vi "Angle-Agle synergy.vi"(11 "Angle for Synergy analysis":dbl[][](array[numeric])) -> (2 "Angle-angle synergygrap":i32[][](array[numeric]), 3 "Angle-angle synergy":dbl[][](array[numeric]))   [LabVIEW 2020]
uses:
  <vilib>/Analysis/NI_AALPro.lvlib
  <vilib>/gmath/NI_Gmath.lvlib
panel:
  out "Angle-angle synergy graph":i32[][](array[numeric])
  out "Angle-angle synergy":dbl[](array[numeric])
  out "r^2":dbl format="%.7g"
  out "correlation coefficient r":dbl format="%.7g"
  out "Elbow flexion - Shoulder graph":i32[](graph)
  out "Elbow flexion - Shoulder extension %":i32
  out "Elbow flexion - Shoulder flexion %":i32
  out "Shoulder flexion - Elbow graph":i32[](graph)
  out "Shoulder flexion - Elbow extension %":i32
  out "Shoulder flexion - Elbow flexion %":i32
  out "Elbow flexion tags":i32[](array[numeric])
  out "Shoulder flexion tags":i32[](array[numeric])
  out "Elbow extension - Shoulder graph":i32[](graph)
  out "Elbow extension - Shoulder flexion %":i32
  out "Elbow extension- Shoulder extension %":i32
  out "Shoulder extension - Elbow graph":i32[](graph)
  out "Shoulder extension - Elbow flexion %":i32
  out "Shoulder extension- Elbow extension %":i32
  out "Shoulder derivative":dbl[](graph)
  out "Shoulder":dbl[](graph)
  out "Shoulder to derivate":dbl[](array[numeric])
  out "Wrist X to graph":dbl[](array[numeric])
  out "Elbow extension tags":i32[](array[numeric])
  out "Shoulder extension tags":i32[](array[numeric])
  out "?":dbl[](graph)
  out "?":dbl[](graph)
  # "Elbow"
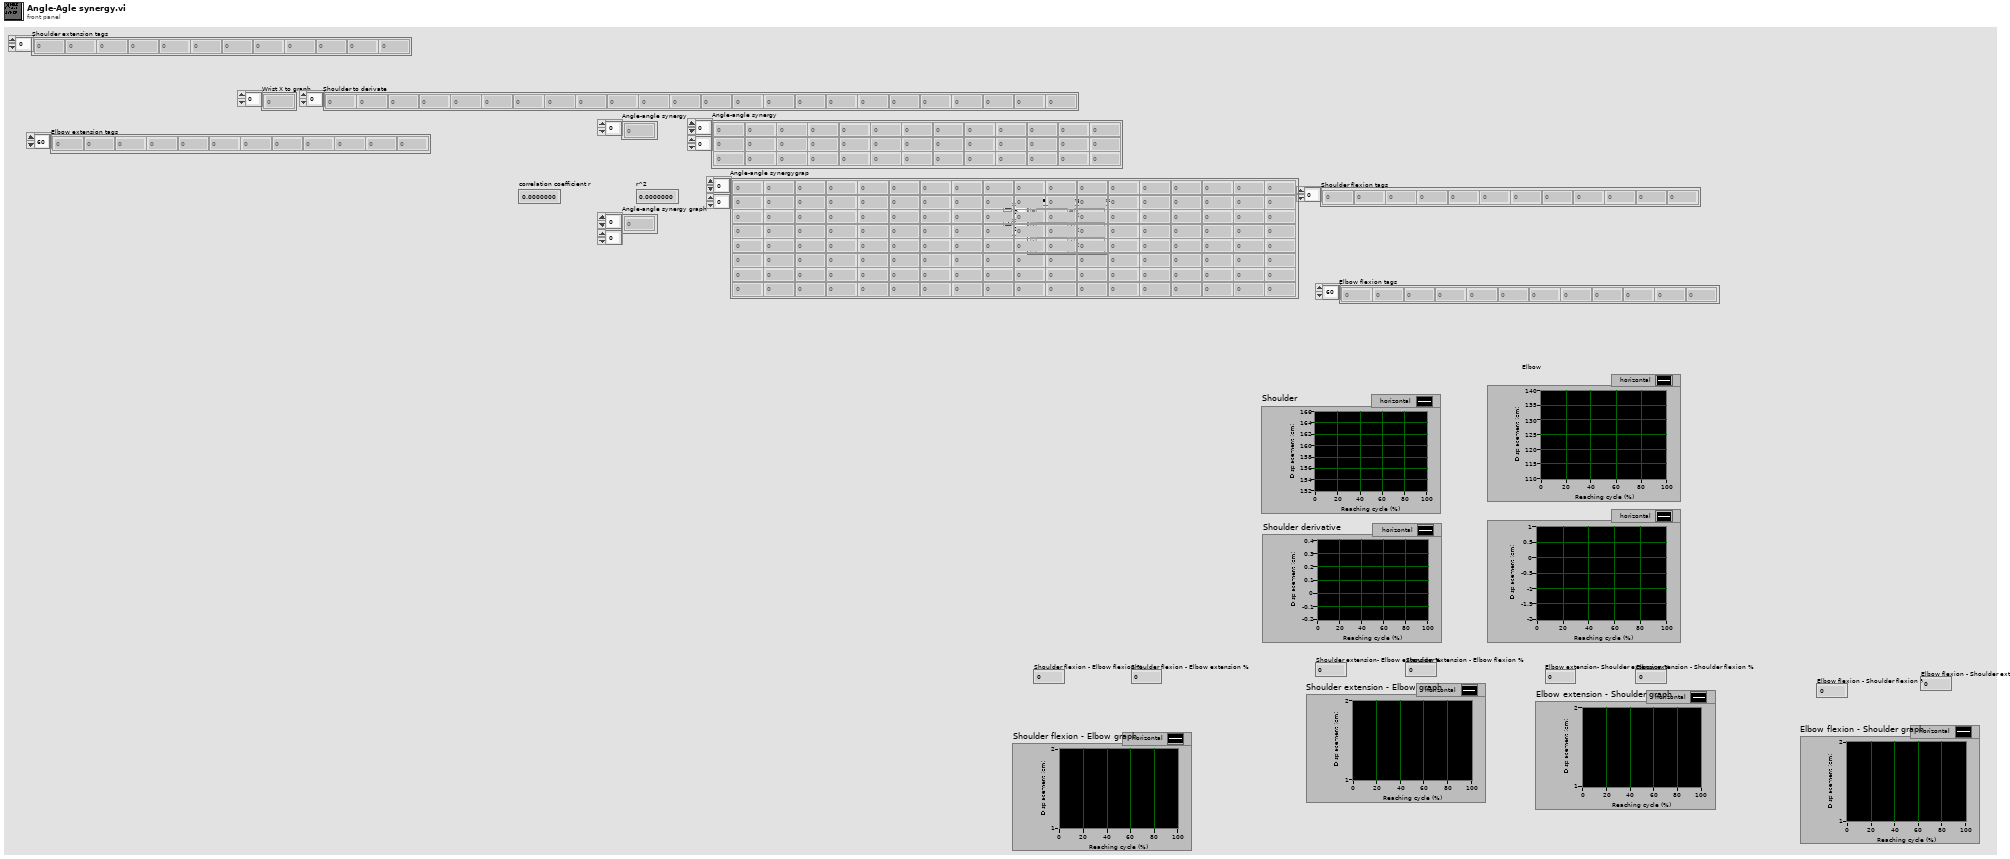
[diagram p1: front panel]
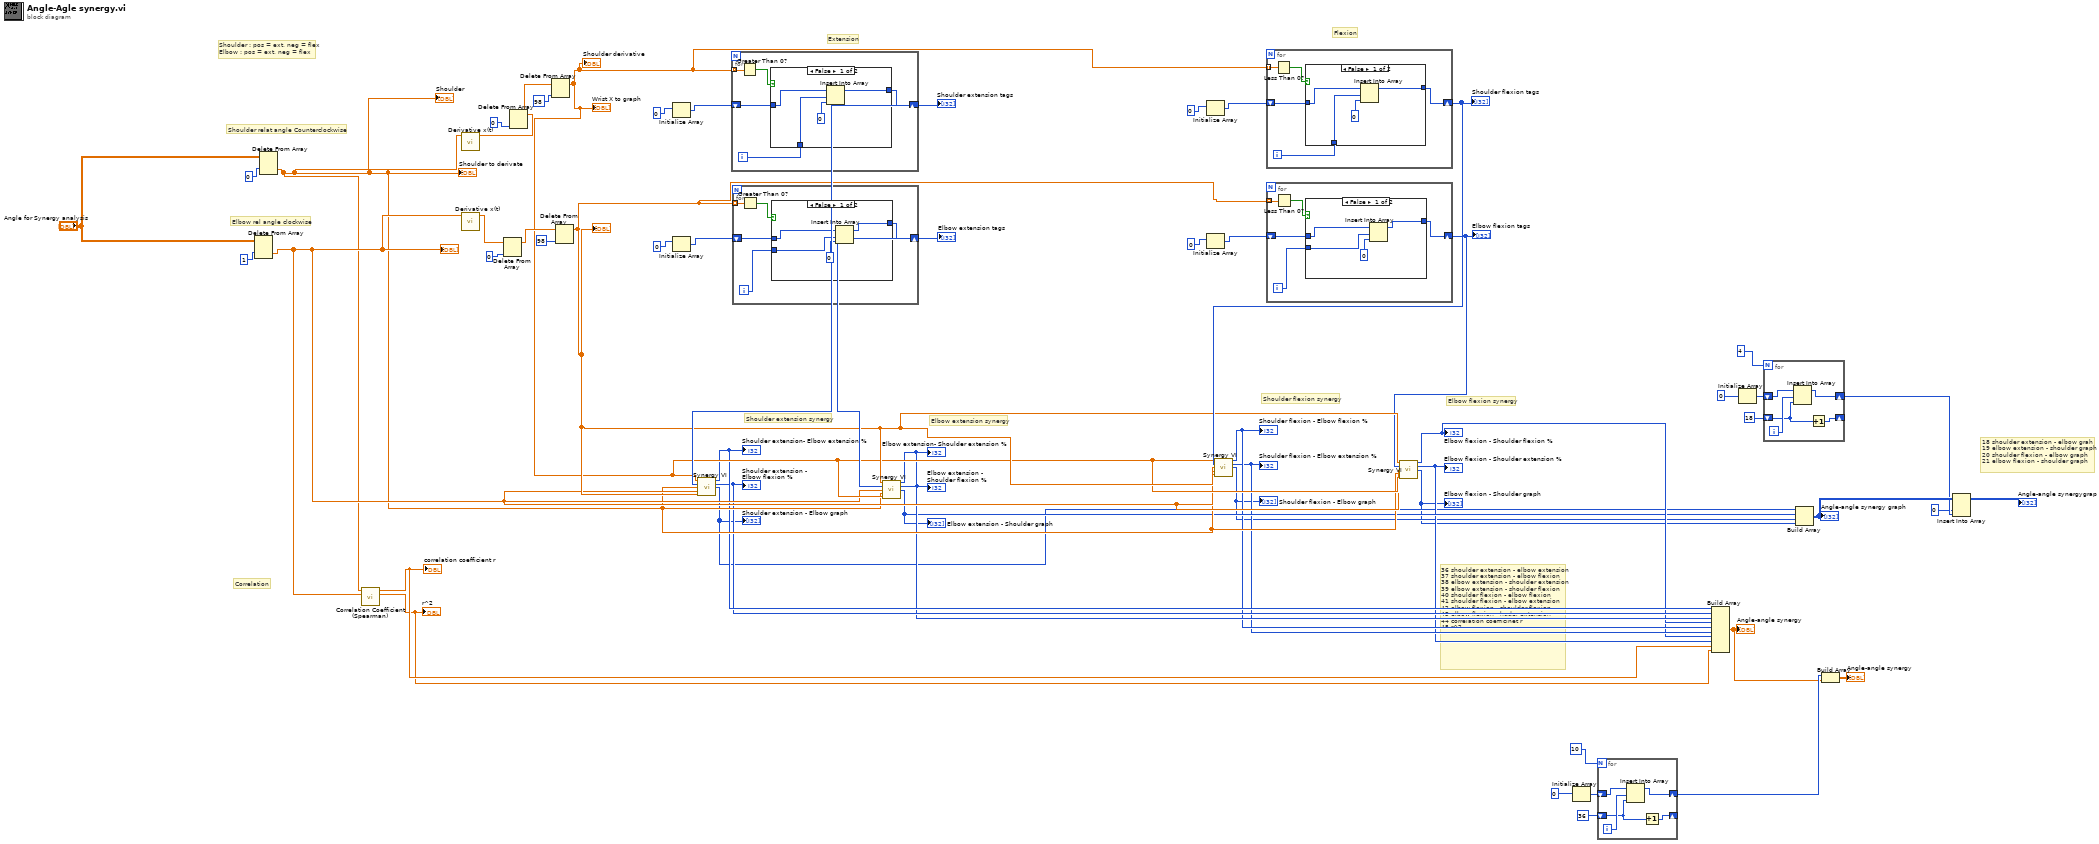
[diagram p0: block diagram]
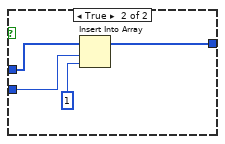
[diagram p2: hidden frame]
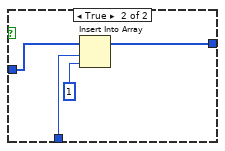
[diagram p3: hidden frame]
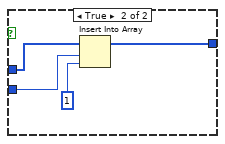
[diagram p4: hidden frame]
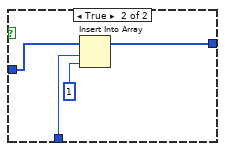
[diagram p5: hidden frame]
diagram:
  # "18 shoulder extension - elbow grah\n19 elbow extension - shoulder graph\n20 shoulder flexion - elbow graph\n21 elbow flexion - shoulder graph"
  # "36 shoulder extension - elbow extension\n37 shoulder extension - elbow flexion\n38 elbow extension - shoulder extension\n39 elbow extension - shoulder flexion\n40 shoulder flexion - elbow flexion\n41 shoulder flexion - elbow extension\n42 elbow flexion - shoulder flexion\n43 elbow flexion - huder extension\n44 correlation coefficinet r\n45 r^2"
  # "Correlation"
  # "Elbow flexion synergy"
  # "Shoulder flexion synergy"
  # "Flexion"
  # "Extension"
  # "Elbow extension synergy"
  # "Shoulder extension synergy"
  # "Shoulder : pos = ext, neg = flex\nElbow : pos = ext, neg = flex"
  # "Elbow rel angle clockwise"
  # "Shoulder relat angle Counterclockwise"
  n1 = Delete From Array(array="Angle for Synergy analysis", index (row)=1) -> (deleted portion=w31:dbl[])  [unwired: 2 in, 1 out]
  "?" <- w31
  n2 = Delete From Array(array="Angle for Synergy analysis", index (row)=0) -> (deleted portion=w30:dbl[])  [unwired: 2 in, 1 out]
  "Shoulder to derivate" <- w30
  "Shoulder" <- w30
  n3 = call <vilib>:"Correlation Coefficient (Spearman).vi"("Y"=w31, "X"=w30) -> ("r^2"=w20:dbl, "correlation coefficient r"=w21:dbl)  [unwired: 8 in]
  "correlation coefficient r" <- w21
  "r^2" <- w20
  n4 = call <vilib>:"Derivative x(t).vi"("X"=w30) -> ("dX/dt"=w56:dbl[])  [unwired: 9 in, 1 out]
  n5 = call <vilib>:"Derivative x(t).vi"("X"=w31) -> ("dX/dt"=w49:dbl[])  [unwired: 9 in, 1 out]
  n6 = Delete From Array(array=w49, index=0) -> (array with subset deleted=w50:dbl[])  [unwired: 1 in, 1 out]
  n7 = Delete From Array(array=w56, index=0) -> (array with subset deleted=w53:dbl[])  [unwired: 1 in, 1 out]
  n8 = Delete From Array(array=w53, index=98) -> (array with subset deleted=w32:dbl[])  [unwired: 1 in, 1 out]
  "Wrist X to graph" <- w32
  "Shoulder derivative" <- w32
  n9 = Delete From Array(array=w50, index=98) -> (array with subset deleted=w34:dbl[])  [unwired: 1 in, 1 out]
  "?" <- w34
  n10 = Initialize Array(0) -> (w47:i32[])  [unwired: 1 in]
  n11 = Initialize Array(0) -> (w45:i32[])  [unwired: 1 in]
  n12 = for {
    tunnel: w32 -> [w61] mode=indexing
    shift-right: [w58] -> w41
    shift-left: w47 -> [w59]
    i -> [w57]
    n13 = Greater Than 0?(x=w61) -> (x > 0?=w60:bool)
    n14 = case shown="False" w60 {
      tunnel: w59 -> [w64 w69]
      tunnel: [w63 w68] -> w58
      tunnel: w57 -> [w62 w66]
      frame False {
        n15 = Insert Into Array(array=w64, index=w62, new element=0) -> (w63:i32[])
      }
      frame True {
        n16 = Insert Into Array(array=w69, index=w66, new element=1) -> (w68:i32[])
      }
    }
  }
  "Shoulder extension tags" <- w41
  n17 = call "Synergy VI.vi"("Wrist X to graph"=w32, "Wrist X Tags"=w41, "Wrist X to derivate"=w30, "Shoulder X to derivate"=w31, "Shoulder X"=w34) -> ("same direction %"=w29:i32, "opposite direction %"=w28:i32, "WristX-ShouldeX graph"=w12:i32[])  [unwired: 8 in]
  "Shoulder extension- Elbow extension %" <- w29
  "Shoulder extension - Elbow flexion %" <- w28
  "Shoulder extension - Elbow graph" <- w12
  n18 = for {
    tunnel: w34 -> [w74] mode=indexing
    shift-right: [w70] -> w40
    shift-left: w45 -> [w72]
    i -> [w71]
    n19 = Greater Than 0?(x=w74) -> (x > 0?=w73:bool)
    n20 = case shown="False" w73 {
      tunnel: w72 -> [w77 w82]
      tunnel: w71 -> [w75 w79]
      tunnel: [w76 w81] -> w70
      frame False {
        n21 = Insert Into Array(array=w77, index=w75, new element=0) -> (w76:i32[])
      }
      frame True {
        n22 = Insert Into Array(array=w82, index=w79, new element=1) -> (w81:i32[])
      }
    }
  }
  "Elbow extension tags" <- w40
  n23 = call "Synergy VI.vi"("Wrist X to graph"=w34, "Wrist X Tags"=w40, "Wrist X to derivate"=w31, "Shoulder X to derivate"=w30, "Shoulder X"=w32) -> ("same direction %"=w27:i32, "opposite direction %"=w26:i32, "WristX-ShouldeX graph"=w11:i32[])  [unwired: 8 in]
  "Elbow extension- Shoulder extension %" <- w27
  "Elbow extension - Shoulder flexion %" <- w26
  "Elbow extension - Shoulder graph" <- w11
  n24 = Initialize Array(0) -> (w38:i32[])  [unwired: 1 in]
  n25 = Initialize Array(0) -> (w36:i32[])  [unwired: 1 in]
  n26 = for {
    tunnel: w32 -> [w87] mode=indexing
    shift-right: [w84] -> w35
    shift-left: w38 -> [w85]
    i -> [w83]
    n27 = Less Than 0?(x=w87) -> (x < 0?=w86:bool)
    n28 = case shown="False" w86 {
      tunnel: w85 -> [w90 w95]
      tunnel: [w89 w94] -> w84
      tunnel: w83 -> [w88 w92]
      frame False {
        n29 = Insert Into Array(array=w90, index=w88, new element=0) -> (w89:i32[])
      }
      frame True {
        n30 = Insert Into Array(array=w95, index=w92, new element=1) -> (w94:i32[])
      }
    }
  }
  "Shoulder flexion tags" <- w35
  n31 = call "Synergy VI.vi"("Wrist X to graph"=w32, "Wrist X Tags"=w35, "Wrist X to derivate"=w30, "Shoulder X to derivate"=w31, "Shoulder X"=w34) -> ("same direction %"=w25:i32, "opposite direction %"=w24:i32, "WristX-ShouldeX graph"=w10:i32[])  [unwired: 8 in]
  "Shoulder flexion - Elbow flexion %" <- w25
  "Shoulder flexion - Elbow extension %" <- w24
  "Shoulder flexion - Elbow graph" <- w10
  n32 = for {
    tunnel: w34 -> [w100] mode=indexing
    shift-right: [w96] -> w33
    shift-left: w36 -> [w98]
    i -> [w97]
    n33 = Less Than 0?(x=w100) -> (x < 0?=w99:bool)
    n34 = case shown="False" w99 {
      tunnel: w98 -> [w103 w108]
      tunnel: w97 -> [w101 w105]
      tunnel: [w102 w107] -> w96
      frame False {
        n35 = Insert Into Array(array=w103, index=w101, new element=0) -> (w102:i32[])
      }
      frame True {
        n36 = Insert Into Array(array=w108, index=w105, new element=1) -> (w107:i32[])
      }
    }
  }
  "Elbow flexion tags" <- w33
  n37 = call "Synergy VI.vi"("Wrist X to graph"=w34, "Wrist X Tags"=w33, "Wrist X to derivate"=w31, "Shoulder X to derivate"=w30, "Shoulder X"=w32) -> ("same direction %"=w23:i32, "opposite direction %"=w22:i32, "WristX-ShouldeX graph"=w9:i32[])  [unwired: 8 in]
  "Elbow flexion - Shoulder flexion %" <- w23
  "Elbow flexion - Shoulder extension %" <- w22
  "Elbow flexion - Shoulder graph" <- w9
  n38 = Initialize Array(0) -> (w17:i32[])  [unwired: 1 in]
  n39 = for {
    N: 10 -> [_]
    shift-right: [w111] -> w15
    shift-left: w17 -> [w112]
    shift-right: [w109] -> _
    shift-left: 36 -> [w110]
    i -> [w113]
    n40 = Insert Into Array(array=w112, index=w113, new element=w110) -> (w111:i32[])
    n41 = Increment(x=w110) -> (x+1=w109:i32)
  }
  n42 = Build Array(w29, w28, w27, w26, w25, w24, w23, w22, w21, w20) -> (w14:dbl[])
  "Angle-angle synergy" <- w14
  n43 = Initialize Array(0) -> (w6:i32[])  [unwired: 1 in]
  n44 = for {
    N: 4 -> [_]
    shift-right: [w116] -> w3
    shift-left: w6 -> [w117]
    shift-right: [w114] -> _
    shift-left: 18 -> [w115]
    i -> [w118]
    n45 = Insert Into Array(array=w117, index=w118, new element=w115) -> (w116:i32[])
    n46 = Increment(x=w115) -> (x+1=w114:i32)
  }
  n47 = Build Array(w12, w11, w10, w9) -> (w4:i32[][])
  "Angle-angle synergy graph" <- w4
  n48 = Build Array(w15, w14) -> (→"Angle-angle synergy":dbl[][])
  n49 = Insert Into Array(array=w4, index (col)=0, new element=w3) -> (→"Angle-angle synergygrap":i32[][])  [unwired: 1 in]
